vi "REV2_Instr.vi"(3 "Parameter":string, 4 "Instruction":T1=1 format="%02x" items=["PING"=1, "READ_STAT"=2, "WRITE_STAT"=3, "READ_CONFIG"=4, "WRITE_CONFIG"=5, "SAVE_CONFIG"=6, "BULK_STAT"=18], 5 "ID":u8 format="%x") -> (2 "Output":string)   [LabVIEW 2016, in "REV_2.lvlib"]
uses:
  REV_2.lvlib
  REV2_Instructions.ctl
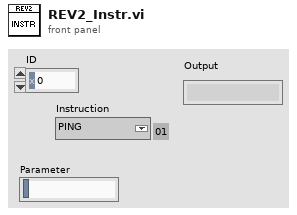
[diagram p1: front panel]
types:
  T1 = typedef "REV_2.lvlib/REV2_Instructions.ctl" = u8
  T2 = enum16{"big-endian, network order", "native, host order", "little-endian"}
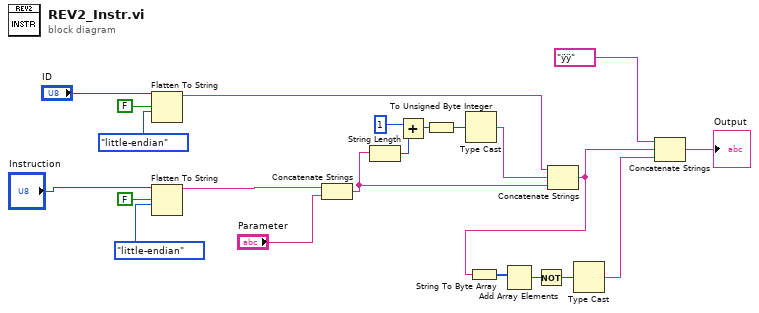
[diagram p0: block diagram]
diagram:
  n1 = Flatten To String(anything="ID", prepend array or string size? (T)=FALSE, byte order (0:big-endian, network order)=T2."little-endian") -> (data string=w2:string)  [unwired: 1 in, 2 out]
  n2 = Flatten To String(anything="Instruction", prepend array or string size? (T)=FALSE, byte order (0:big-endian, network order)=T2."little-endian") -> (data string=w6:string)  [unwired: 1 in, 2 out]
  n3 = Concatenate Strings(w6, "Parameter") -> (w10:string)
  n4 = String Length(string=w10) -> (length=w16:i32)
  n5 = Add(x=1, y=w16) -> (x+y=w18:i32)
  n6 = To Unsigned Byte Integer(number=w18) -> (unsigned 8bit integer=w19:u8)
  n7 = Type Cast(x=w19) -> (*(type *) &x=w20:string)  [unwired: 1 in]
  n8 = Concatenate Strings(w2, w20, w10) -> (w21:string)
  n9 = String To Byte Array(string=w21) -> (unsigned byte array=w13:u8[])
  n10 = Add Array Elements(numeric array=w13) -> (sum=w15:u8)
  n11 = Not(x=w15) -> (.not. x?=w14:u8)
  n12 = Type Cast(x=w14) -> (*(type *) &x=w22:string)  [unwired: 1 in]
  n13 = Concatenate Strings("ÿÿ" ("string"), w21, w22) -> (→"Output":string)
